vi "Dashboard IP Camera Loop.vi"(9 "Camera IP":string, 10 "Close?":bool, 11 "Refnum in":T1) -> (0 "error out":errorcluster, 2 "Active":bool, 3 "Refnum out":T1, 4 "FPS":dbl, 5 "Bandwidth (Mbps)":dbl)   [LabVIEW 2015]
uses:
  <vilib>/vision/Image Controls.llb/IMAQ Image.ctl
  <vilib>/Rock Robotics/WPI/Camera/WPI_CameraSettings Read MJPG.ctl
  <vilib>/Rock Robotics/WPI/Camera/WPI_CameraImageSize.ctl
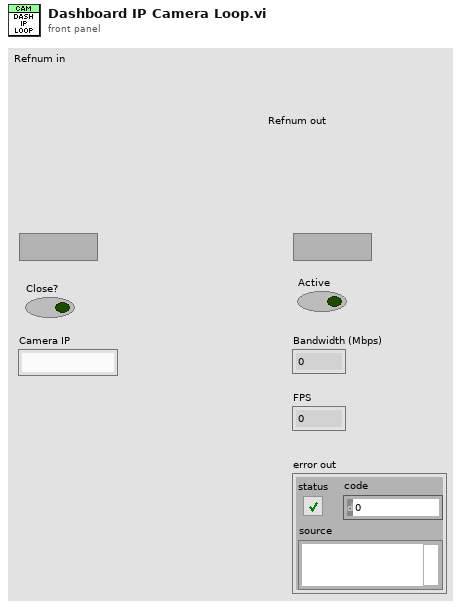
[diagram p1: front panel]
types:
  T1 = typedef "IMAQ Image.ctl" = refnum<image>
  T2 = typedef "WPI_CameraSettings Read MJPG.ctl" = cluster{"fps":i32, "compression":i32, "Image Size":T3}
  T3 = typedef "WPI_CameraImageSize.ctl" = enum16{"640x480", "320x240", "160x120", "Custom"}
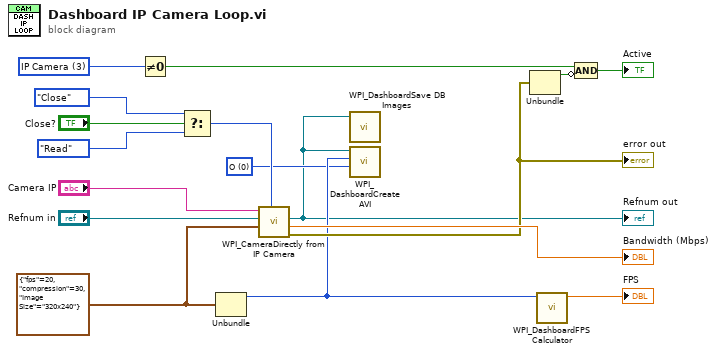
[diagram p0: block diagram]
diagram:
  w2 = u16 0 items=["O", "*", "Open Playback Panel"] ("Recording")
  w16 = T2 {"fps"=20, "compression"=30, "Image Size"=enum."320x240"} ("Camera Settings")
  w5 = u16 3 items=["Camera Off", "USB Camera SW", "USB Camera HW", "IP Camera"] ("Camera Mode")
  n1 = Not Equal To 0?(x=w5) -> (x != 0?=w6:bool)
  n2 = Select(t=enum16{"Read", "Reopen", "Close"}."Close" ("Operation"), s="Close?", f=enum16{"Read", "Reopen", "Close"}."Read" ("Operation")) -> (s? t:f=w13:enum16{"Read", "Reopen", "Close"})
  n3 = Unbundle(w16) -> ("fps"=w3:i32)  [unwired: 2 out]
  n4 = call <vilib>:"WPI_CameraDirectly from IP Camera.vi"("Operation"=w13, "Camera Settings"=w16, "Image"="Refnum in", "address"="Camera IP") -> ("error out"=w7:errorcluster, "Bandwidth (Mbps)"=→"Bandwidth (Mbps)":dbl, "Image Out"=w1:T1)  [unwired: 5 in]
  "Refnum out" <- w1
  "error out" <- w7
  n5 = call <vilib>:"WPI_DashboardSave DB Images.vi"("Image"=w1) -> ()  [unwired: 3 in]
  n6 = call <vilib>:"WPI_DashboardCreate AVI.vi"("Recording"=w2, "frames per seconds"=w3, "Image"=w1) -> ()  [unwired: 9 in]
  n7 = Unbundle(w7) -> ("status"=w14:bool)  [unwired: 2 out]
  n8 = call <vilib>:"WPI_DashboardFPS Calculator.vi"("Average Count"=w3) -> ("fps"=→"FPS":dbl)  [unwired: 10 in]
  n9 = Compound Arithmetic op=AND(w6, invert w14) -> (→"Active":bool)
